vi "Create.vi"(8 "error in (no error)":errorcluster, 11 "SHD in":refnum<class "SHINI SHD.lvclass">) -> (0 "error out":errorcluster, 3 "SHD out":refnum<class "SHINI SHD.lvclass">)   [LabVIEW 2021, in "SHINI SHD.lvclass"]
uses:
  SHINI SHD.lvclass
  D:/my_projects/projects/21/Master CR/Master CR.lvclass
  Master CR.lvclass/Master CR.ctl
  ET7000/TCP/TCP.lvclass
  SHINI SHD.lvclass/SHINI SHD.ctl
  Master CR.lvclass
  Data Model/SHD Data Model/SHD Data Model.lvclass
  D:/my_projects/projects/21/Master CR/Data Model/ICPCON ET7000 Data Model/ICPCON ET Data Model.lvclass
  D:/my_projects/projects/21/Modbus_v121c/Data Model/Device Data Model.lvclass
  D:/my_projects/projects/21/Master CR/Data Model/SHD Data Model/SHD Data Model.lvclass
  D:/my_projects/projects/21/Master CR/Devices/ET7000/TCP/TCP.lvclass
  D:/my_projects/projects/21/Master CR/Devices/SHINI/SHD/SHINI SHD.lvclass
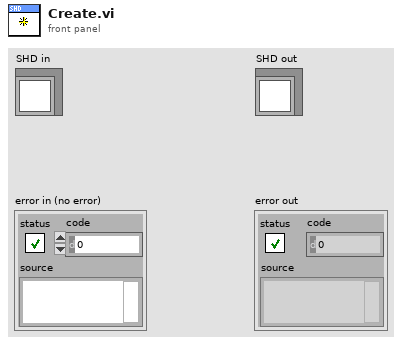
[diagram p1: front panel]
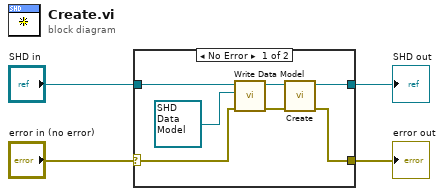
[diagram p0: block diagram]
diagram:
  n1 = case shown="No Error" "error in (no error)" {
    selector: "error in (no error)" -> [w5 w12]
    tunnel: [w9 w12] -> w1
    tunnel: [w10 w13] -> w2
    tunnel: "SHD in" -> [w11 w13]
    frame No Error {
      n2 = call "Write Data Model.vi"("error in (no error)"=w5, "Data Model"=refnum<class "SHD Data Model.lvclass"> refnum ("Modbus API:Device Data Model"), "Master CR in"=w11) -> ("error out"=w8:errorcluster, "Master CR out"=w7:refnum<class "SHINI SHD.lvclass">)  [unwired: 7 in]
      n3 = call-parent "Create.vi"("error in (no error)"=w8, "TCP in"=w7) -> ("error out"=w9:errorcluster, "TCP out"=w10:refnum<class "SHINI SHD.lvclass">)  [unwired: 8 in]
    }
    frame Error {
    }
  }
  "error out" <- w1
  "SHD out" <- w2
